vi "Test API Throws Error lvproj not Found.vi"(8 "error in (no error)":errorcluster, 11 "API Test in":refnum<class "API Test.lvclass">) -> (0 "error out":errorcluster, 3 "API Test out":refnum<class "API Test.lvclass">)   [LabVIEW 2020, in "LUnit Tests.lvlib" / "API Test.lvclass"]
uses:
  API Test.lvclass
  source/Framework/Execution API/Execution API.lvclass
  <vilib>/Astemes/LUnit/Test Case.lvclass
  C:/Program Files (x86)/National Instruments/LabVIEW 2021/vi.lib/Astemes/LUnit/Test Case.lvclass
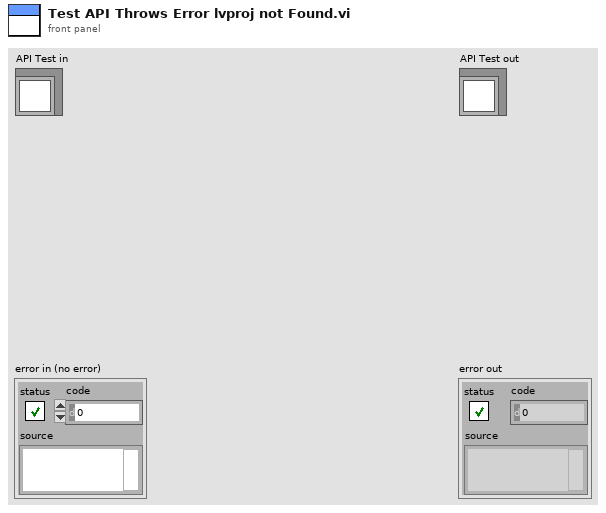
[diagram p1: front panel]
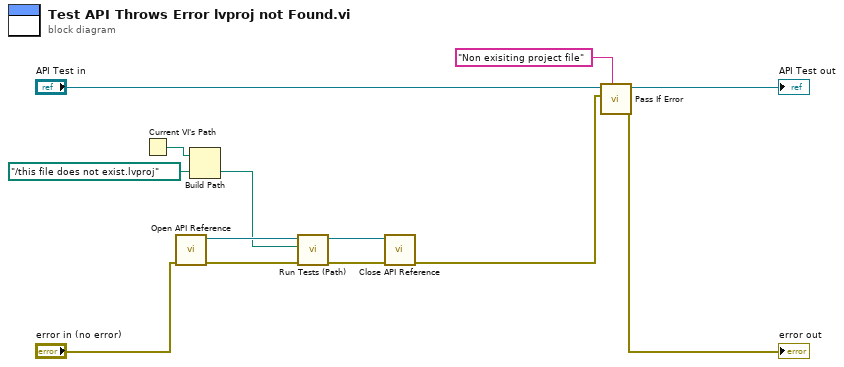
[diagram p0: block diagram]
diagram:
  n1 = Current VI's Path() -> (path=w2:path)
  n2 = call "Open API Reference.vi"("error in (no error)"="error in (no error)") -> ("error out"=w12:errorcluster, "Execution API out"=w13:refnum<class "Execution API.lvclass">)  [unwired: 9 in]
  n3 = Build Path(base path=w2, name or relative path=path "../this file does not exist.lvproj") -> (appended path=w3:path)
  n4 = call "Run Tests (Path).vi"("error in (no error)"=w12, "Project or Class Path"=w3, "Execution API In"=w13) -> ("error out"=w11:errorcluster, "Execution API Out"=w10:refnum<class "Execution API.lvclass">)  [unwired: 7 in]
  n5 = call "Close API Reference.vi"("error in (no error)"=w11, "Execution API in"=w10) -> ("error out"=w6:errorcluster)  [unwired: 9 in]
  n6 = call <vilib>:"Pass If Error.vi"("Description"="Non exisiting project file", "Assert error"=w6, "LUnit Test Case In"="API Test in") -> ("error out"=→"error out":errorcluster, "LUnit Test Case Out"=→"API Test out":refnum<class "API Test.lvclass">)  [unwired: 7 in]
